vi "Ej_10_Inicializar_Variables.vi"() -> ()   [LabVIEW 2021]
panel:
  in  "stop":bool
  out "Indicador contraseña":string
  in  "Contraseña":string
  in  "Nombre":string
  out "Indicador nombre":string
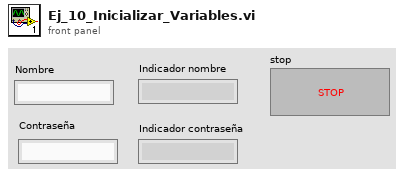
[diagram p1: front panel]
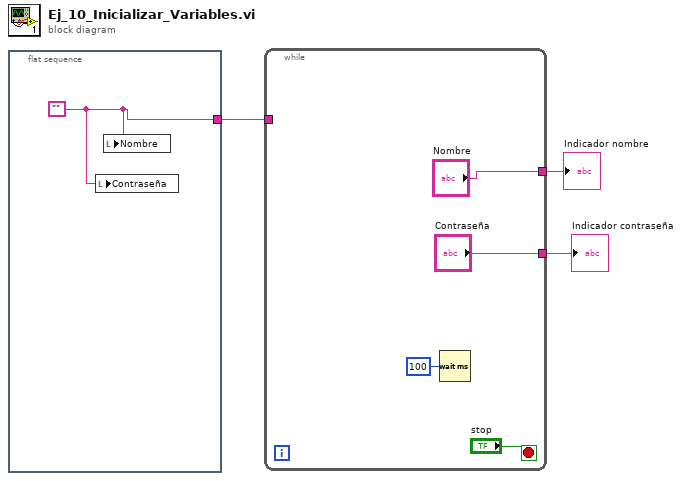
[diagram p0: block diagram]
diagram:
  n1 = flat-sequence {
    tunnel: [w4] -> w1
    frame #0 {
      w4 = ""
      n2 = local write "Contraseña"(w4) -> ()
      n3 = local write "Nombre"(w4) -> ()
    }
  }
  n4 = while {
    tunnel: ["Nombre"] -> w3
    tunnel: ["Contraseña"] -> w2
    tunnel: w1 -> [_]
    stop <- "stop" stop-if-true
    n5 = Wait (ms)(milliseconds to wait=u32 100) -> ()  [unwired: 1 out]
  }
  "Indicador contraseña" <- w2
  "Indicador nombre" <- w3
